vi "R2R-Controller.vi"(4 "Custom Controller Inputs":T1, 6 "Gain Configuration":T2={"PID Gains"={"proportional gain (Kc)"=1.0, "integral gain (Kc*Ts/Ti)"=0.0, "derivative gain (Kc*Td/Ts)"=0.0}, "Output Range"={"output high"=10.0, "output low"=-10.0}}, 7 "Reset Integrator":bool, 8 "X (Raw Analog V)":fxp<+,18,3>, 9 "F (Raw Analog V)":fxp<+,18,3>, 10 "X* (mm)":fxp<+/-,16,7>, 11 "F* (N)":fxp<+/-,16,7>) -> (0 "Xmeas (mm)":fxp<+/-,35,12>, 1 "Fmeas (N)":fxp<+,39,10>, 2 "V*(V)":fxp<+/-,53,13> format="%.6f", 3 "PWM Duty Cycle":i16, 5 "Duty Cycle Output":i16)   [LabVIEW 2013]
uses:
  controls/Control Configuration.ctl
  controls/Custom Controller Inputs.ctl
  <vilib>/rvi/Analysis/measure/butterworth/XNode/niFpgaButterworthFilter.xnode
  <vilib>/addons/control/pid/fpga.llb/XNode/niFpgaPID.xnode
panel:
  out "Y*'":fxp<+/-,36,35>
  out "Y*":fxp<+/-,64,31> format="%.41g"
  in  "K_PosSense (mm/Volt)":fxp<+,12,4>=10.0
  out "deltaX*":fxp<+/-,49,21> format="%.34g"
  out "Ferr (N)":fxp<+/-,40,11>
  in  "K_PWM (Counts/Volt)":fxp<+,16,7>=83.33203125
  in  "Ra (Armature Resistance) (Ohms)":fxp<+/-,7,7>=60.0
  out "I* Current Command (A)":fxp<+/-,48,8>
  in  "Force Sensor Gain (N/V)":fxp<+,20,6>=53.02703857421875
  in  "L12 Gain (mA/N)":fxp<+,16,2>=2.29180908203125
  in  "L12 Offset (mA)":fxp<+,18,4>=12.9949951171875
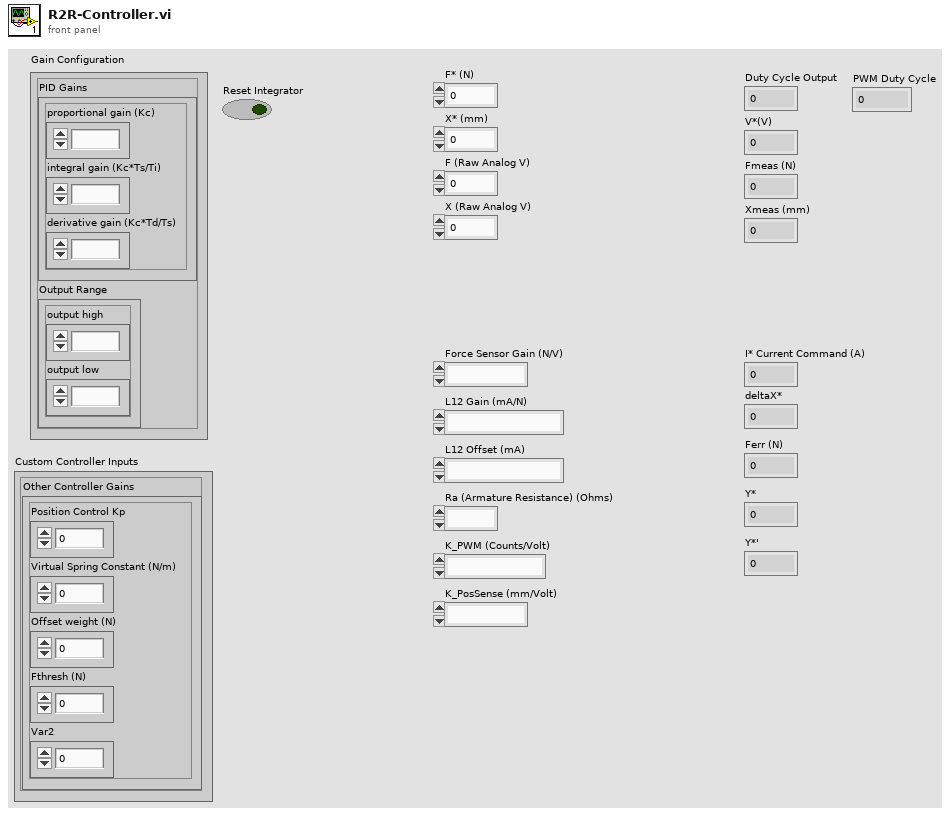
[diagram p1: front panel]
types:
  T1 = typedef "Custom Controller Inputs.ctl" = cluster{"Other Controller Gains":cluster{"Position Control Kp":fxp<+/-,16,8>, "Virtual Spring Constant (N/m)":fxp<+,16,12>, "Offset weight (N)":fxp<+/-,16,8>, "Fthresh (N)":fxp<+/-,16,5>, "Var2":fxp<+/-,16,5>}}
  T2 = typedef "Control Configuration.ctl" = cluster{"PID Gains":cluster{"proportional gain (Kc)":fxp<+/-,16,8>, "integral gain (Kc*Ts/Ti)":fxp<+/-,16,8>, "derivative gain (Kc*Td/Ts)":fxp<+/-,16,8>}, "Output Range":cluster{"output high":fxp<+/-,16,7>, "output low":fxp<+/-,16,7>}}
  T3 = cluster{"Position Control Kp":fxp<+/-,16,8>, "Virtual Spring Constant (N/m)":fxp<+,16,12>, "Offset weight (N)":fxp<+/-,16,8>, "Fthresh (N)":fxp<+/-,16,5>, "Var2":fxp<+/-,16,5>}
  T4 = cluster{"proportional gain (Kc)":fxp<+/-,16,8>, "integral gain (Kc*Ts/Ti)":fxp<+/-,16,8>, "derivative gain (Kc*Td/Ts)":fxp<+/-,16,8>}
  T5 = cluster{"output high":fxp<+/-,16,7>, "output low":fxp<+/-,16,7>}
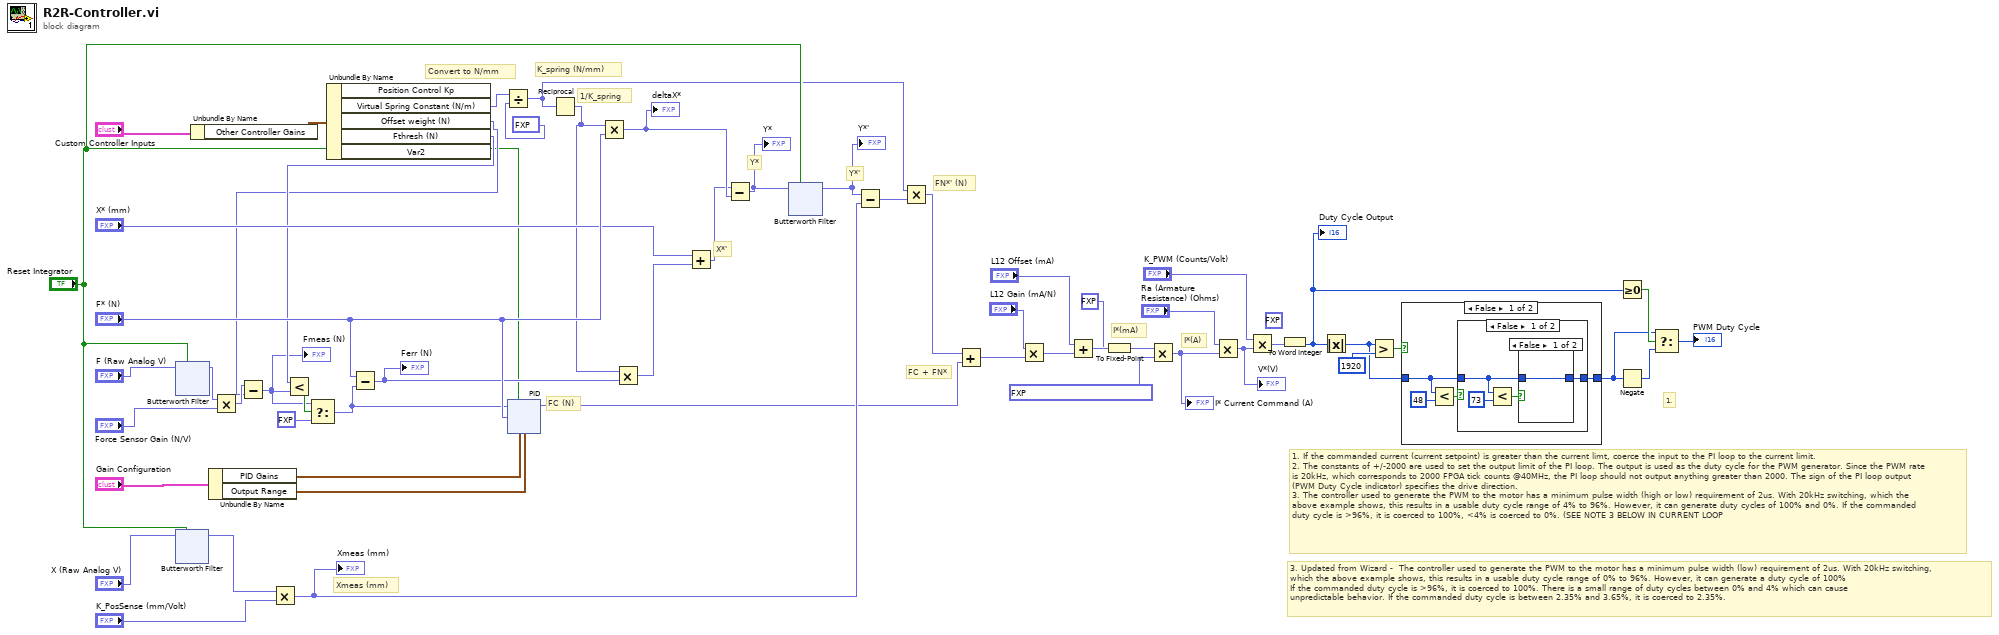
[diagram p0: block diagram]
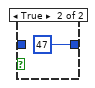
[diagram p2: hidden frame]
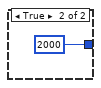
[diagram p4: hidden frame]
diagram:
  (unwired) fxp<+/-,16,16> 0.0 ("fixed-point type")
  # "FC + FN*"
  # "K_spring (N/mm)"
  # "Convert to N/mm"
  # "1. If the commanded current (current setpoint) is greater than the current limt, coerce the input to the PI loop to the current limit.\n2. The constants of +/-2000 are used to set the output limit of the PI loop. The output is used as the duty cycle for the PWM generator. Since the PWM rate is 20kHz, which corresponds to 2000 FPGA tick counts @40MHz, the PI loop should not output anything greater than 2000. The sign of the PI loop output (PWM Duty Cycle indicator) specifies the drive direction.\n3. The controller used to generate the PWM to the motor has a minimum pulse width (high or low) requirement of 2us. With 20kHz switching, which the above example shows, this results in a usable duty cycle range of 4% to 96%. However, it can generate duty cycles of 100% and 0%. If the commanded duty cycle is >96%, it is coerced to 100%, <4% is coerced to 0%. (SEE NOTE 3 BELOW IN CURRENT LOOP"
  # "3. Updated from Wizard -  The controller used to generate the PWM to the motor has a minimum pulse width (low) requirement of 2us. With 20kHz switching, which the above example shows, this results in a usable duty cycle range of 0% to 96%. However, it can generate a duty cycle of 100%\nIf the commanded duty cycle is >96%, it is coerced to 100%. There is a small range of duty cycles between 0% and 4% which can cause\nunpredictable behavior. If the commanded duty cycle is between 2.35% and 3.65%, it is coerced to 2.35%."
  # "1."
  # "Y*'"
  # "I*(A)"
  # "I*(mA)"
  # "FC (N)"
  # "FN*' (N)"
  # "Xmeas (mm)"
  # "Y*"
  # "X*'"
  # "1/K_spring"
  n1 = xnode "Butterworth Filter"("input data"="X (Raw Analog V)", "reset"="Reset Integrator") -> ("output data"=w6:fxp<+/-,23,8>)  [unwired: 1 in]
  n2 = xnode "Butterworth Filter"("input data"="F (Raw Analog V)", "reset"="Reset Integrator") -> ("output data"=w9:fxp<+/-,23,8>)  [unwired: 1 in]
  n3 = Unbundle By Name("Custom Controller Inputs") -> ("Other Controller Gains"=w51:T3)
  n4 = Unbundle By Name("Gain Configuration") -> ("PID Gains"=w55:T4, "Output Range"=w54:T5)
  n5 = Multiply(x=w9, y="Force Sensor Gain (N/V)") -> (x*y=w12:fxp<+/-,43,14>)
  n6 = Multiply(x=w6, y="K_PosSense (mm/Volt)") -> (x*y=w43:fxp<+/-,35,12>)
  "Xmeas (mm)" <- w43
  n7 = Unbundle By Name(w51) -> ("Virtual Spring Constant (N/m)"=w1:fxp<+,16,12>, "Offset weight (N)"=w11:fxp<+/-,16,8>, "Fthresh (N)"=w13:fxp<+/-,16,5>)  [unwired: 2 out]
  n8 = Subtract(x=w12, y=w11) -> (x-y=w10:fxp<+/-,44,15>)
  "Fmeas (N)" <- w10
  n9 = Less?(x=w13, y=w10) -> (x < y?=w19:bool)
  n10 = Select(t=w10, s=w19, f=fxp<+,38,9> 0.0) -> (s? t:f=w17:fxp<+/-,44,15>)
  n11 = Subtract(x="F* (N)", y=w17) -> (x-y=w49:fxp<+/-,44,15>)
  "Ferr (N)" <- w49
  n12 = Divide(x=w1, y=fxp<+,17,10> 1000.0) -> (x/y=w3:fxp<+,33,19>)
  n13 = xnode "PID"("process variable"=w17, "reset?"="Reset Integrator", "setpoint"="F* (N)", "PID gains"=w55, "output range"=w54) -> ("output"=w40:fxp<+/-,16,15>)
  n14 = Reciprocal(x=w3) -> (1/x=w4:fxp<+,34,15>)
  n15 = Multiply(x=w4, y="F* (N)") -> (x*y=w46:fxp<+/-,49,21>)
  "deltaX*" <- w46
  n16 = Multiply(x=w4, y=w49) -> (x*y=w47:fxp<+/-,64,29>)
  n17 = Add(x="X* (mm)", y=w47) -> (x+y=w45:fxp<+/-,64,30>)
  n18 = Subtract(x=w45, y=w46) -> (x-y=w31:fxp<+/-,64,31>)
  "Y*" <- w31
  n19 = xnode "Butterworth Filter"("input data"=w31, "reset"="Reset Integrator") -> ("output data"=w30:fxp<+/-,36,35>)  [unwired: 1 in]
  "Y*'" <- w30
  n20 = Subtract(x=w30, y=w43) -> (x-y=w42:fxp<+/-,59,36>)
  n21 = Multiply(x=w3, y=w42) -> (x*y=w41:fxp<+/-,64,54>)
  n22 = Add(x=w41, y=w40) -> (x+y=w38:fxp<+/-,64,55>)
  n23 = Multiply(x="L12 Gain (mA/N)", y=w38) -> (x*y=w37:fxp<+/-,64,57>)
  n24 = Add(x="L12 Offset (mA)", y=w37) -> (x+y=w22:fxp<+/-,64,58>)
  n25 = To Fixed-Point(fixed-point type=fxp<+/-,32,16> 0.0, number=w22) -> (fixed-point=w20:fxp<+/-,32,16>)
  n26 = Multiply(x=w20, y=fxp<+/-,16,-8> 0.0009999871253967285) -> (x*y=w14:fxp<+/-,48,8>)
  "I* Current Command (A)" <- w14
  n27 = Multiply(x="Ra (Armature Resistance) (Ohms)", y=w14) -> (x*y=w33:fxp<+/-,53,13>)
  "V*(V)" <- w33
  n28 = Multiply(x="K_PWM (Counts/Volt)", y=w33) -> (x*y=w16:fxp<+/-,64,20>)
  n29 = To Word Integer(number=w16) -> (16bit integer=w15:i16)
  "Duty Cycle Output" <- w15
  n30 = Absolute Value(x=w15) -> (abs(x)=w24:i16)
  n31 = Greater?(x=w24, y=i16 1920 ("upper limit")) -> (0:w26:bool)
  n32 = case shown="False" w26 {
    tunnel: [w59 i16 2000 ("upper limit")] -> w25
    tunnel: w24 -> [w57 _]
    frame False {
      n33 = Less?(x=w57, y=i16 48 ("lower limit")) -> (x < y?=w58:bool)
      n34 = case shown="False" w58 {
        tunnel: [w61 w67] -> w59
        tunnel: w57 -> [w62 w67]
        frame False {
          n35 = Less?(x=w62, y=i16 73 ("lower limit")) -> (x < y?=w63:bool)
          n36 = case shown="False" w63 {
            tunnel: w62 -> [w65 _]
            tunnel: [w65 i16 47 ("lower limit")] -> w61
            frame False {
            }
            frame True {
            }
          }
        }
        frame True {
        }
      }
    }
    frame True {
    }
  }
  n37 = Greater Or Equal To 0?(x=w15) -> (x >= 0?=w29:bool)
  n38 = Negate(x=w25) -> (-x=w28:i16)
  n39 = Select(t=w25, s=w29, f=w28) -> (s? t:f=→"PWM Duty Cycle":i16)
